vi "Agilent_Save_Array.vi"(2 "Error Array In":errorcluster[](array[cluster]), 3 "Agilent Download":bool=TRUE, 4 "Agilent Array In":T1[](array[typedef]), 5 "File Path":path) -> (0 "Error Array Out":errorcluster[](array[cluster]), 1 "Agilent Array Out":T1[](array[typedef]))   [LabVIEW 2020]
uses:
  AgilentTotalCluster.ctl
  AgilentControl.ctl
  Channel Config.ctl
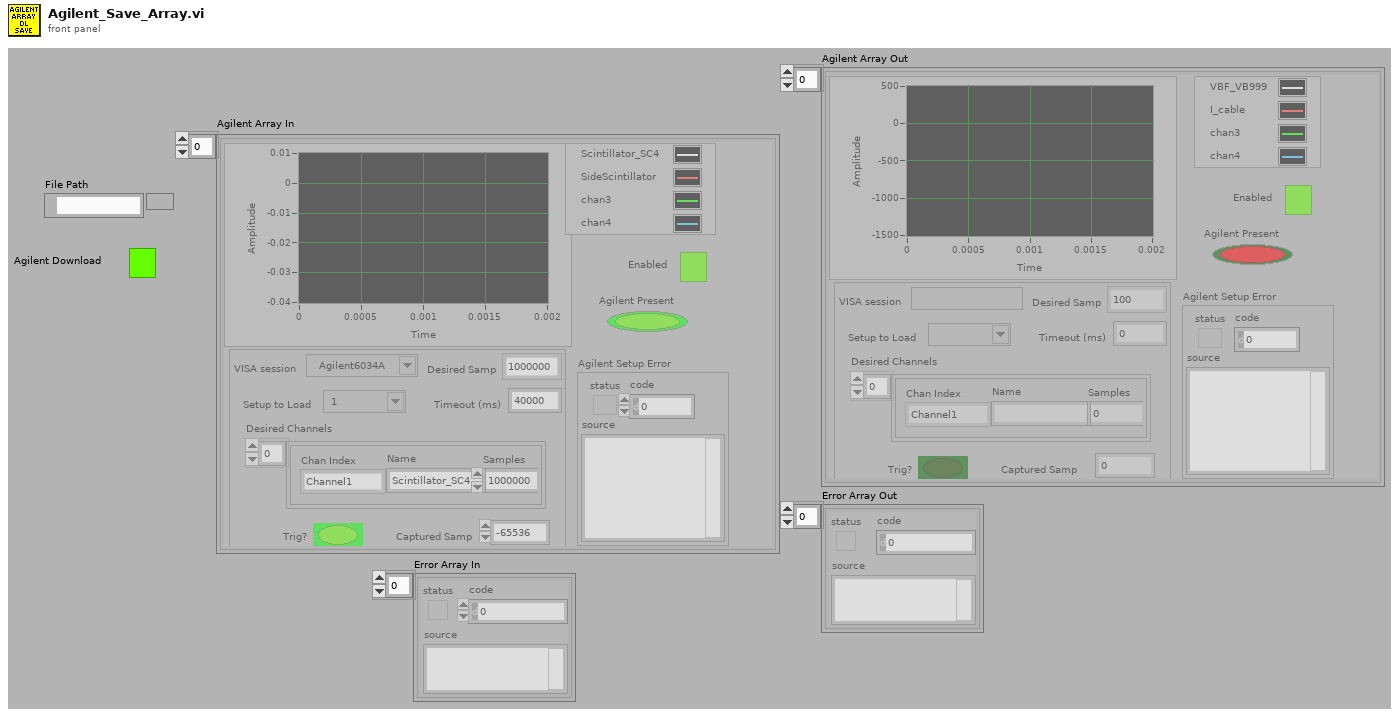
[diagram p1: front panel]
types:
  T1 = typedef "AgilentTotalCluster.ctl" = cluster{"Agilent Graph":waveform(dbl)[], "Agilent Control":T2, "Agilent Setup Error":errorcluster, "Agilent Present":bool, "Enabled":bool}
  T2 = typedef "AgilentControl.ctl" = cluster{"Trig?":bool, "VISA session":refnum<visa-resource-name>, "Setup to Load":string, "Timeout (ms)":u32, "Desired Samp":enum32{"100", "250", "500", "1000", "2000", "5000", "10000", "20000", "50000", "100000", "200000", "500000", "1000000", "2000000", "4000000", "8000000"}, "Captured Samp":i32, "Desired Channels":T3[]}
  T3 = typedef "Channel Config.ctl" = cluster{"Chan Index":enum16{"Channel1", "Channel2", "Channel3", "Channel4", "MATH"}, "Name":string, "Samples":i32}
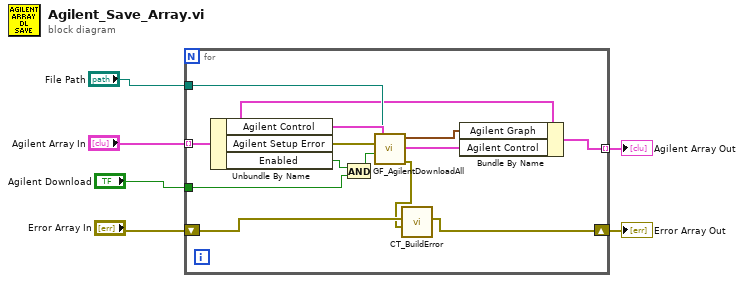
[diagram p0: block diagram]
diagram:
  n1 = for {
    tunnel: "Agilent Array In" -> [w15] mode=indexing
    tunnel: "File Path" -> [w18]
    tunnel: "Agilent Download" -> [w8]
    shift-right: [w16] -> w1
    shift-left: "Error Array In" -> [w17]
    tunnel: [w13] -> w2 mode=indexing
    n2 = Unbundle By Name(w15) -> ("Agilent Control"=w19:T2, "Agilent Setup Error"=w10:errorcluster, "Enabled"=w9:bool)
    n3 = And(x=w9, y=w8) -> (x .and. y?=w7:bool)
    n4 = call "GF_AgilentDownloadAll.vi"("Error In"=w10, "Agilent Download"=w7, "Agilent Cluster In"=w19, "File Path"=w18) -> ("error out"=w11:errorcluster, "Agilent Cluster Out"=w14:T2, "Agilent Scintillator Scope Graph"=w12:waveform(dbl)[])  [unwired: 1 in]
    n5 = call "CT_BuildError.vi"("New Error"=w11, "Error Array In"=w17) -> ("Error Array Out"=w16:errorcluster[])  [unwired: 9 in]
    n6 = Bundle By Name(cluster=w15, "Agilent Graph"=w12, "Agilent Control"=w14) -> (w13:T1)
  }
  "Agilent Array Out" <- w2
  "Error Array Out" <- w1
